vi "Register Group.vi"(8 "error in (no error)":errorcluster, 10 "Group":refnum<class "Group.lvclass">, 11 "RemoteDataService in":refnum<class "RemoteDataService.lvclass">) -> (0 "error out":errorcluster, 3 "RemoteDataService out":refnum<class "RemoteDataService.lvclass">)   [LabVIEW 2020, in "Vecto.lvlib" / "RemoteDataService.lvclass"]
uses:
  RemoteDataService.lvclass
  Group/Group.lvclass
  Register Group Data.ctl
  RemoteDataService.lvclass/RemoteDataService.ctl
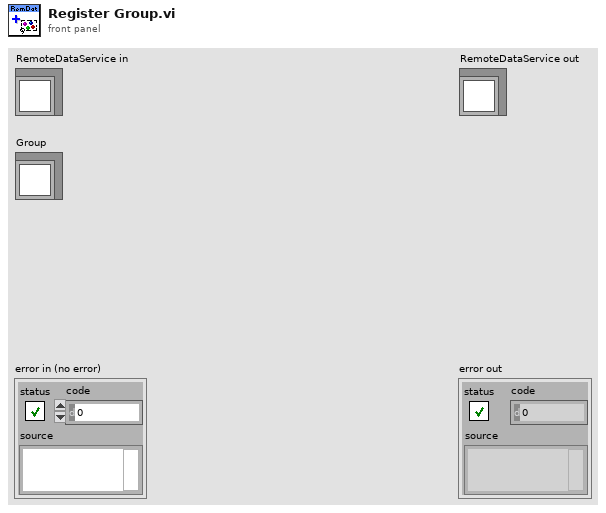
[diagram p1: front panel]
types:
  T1 = typedef "Vecto.lvlib/RemoteDataService.lvclass/Register Group Data.ctl" = cluster{"Group":refnum<class "Group.lvclass">}
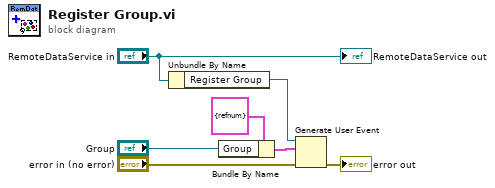
[diagram p0: block diagram]
diagram:
  n1 = Unbundle By Name("RemoteDataService in") -> ("Register Group"=w6:refnum<user-event>)
  n2 = Bundle By Name(cluster=T1 {"Group"=refnum} ("event data"), "Group"="Group") -> (w4:T1)
  n3 = Generate User Event(user event=w6, event data cluster=w4, error in="error in (no error)") -> (error out=→"error out":errorcluster)  [unwired: 1 in, 1 out]
  "RemoteDataService out" <- "RemoteDataService in"
